vi "Write Log File.vi"(6 "time":dbl format="%.3fs", 7 "error? (F)":bool, 8 "error in (no error)":errorcluster, 9 "line text":string, 10 "line tag":string, 11 "file refnum in":refnum<file>) -> (0 "error out":errorcluster, 3 "file refnum out":refnum<file>)   [LabVIEW 2017, in "DSF Core.lvlib" / "Logging Thread.lvclass"]
uses:
  Logging Thread.lvclass
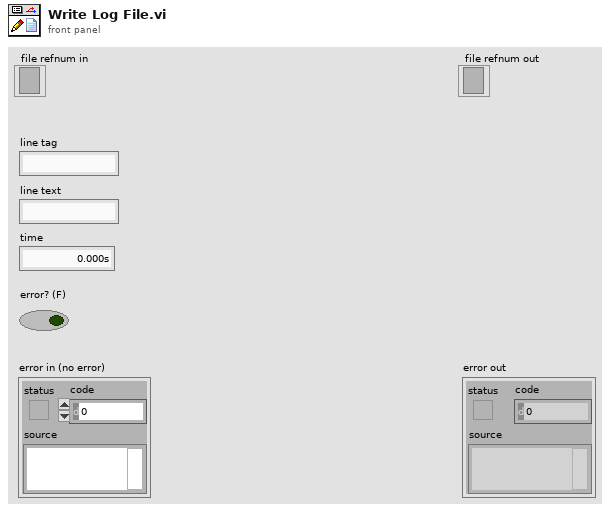
[diagram p1: front panel]
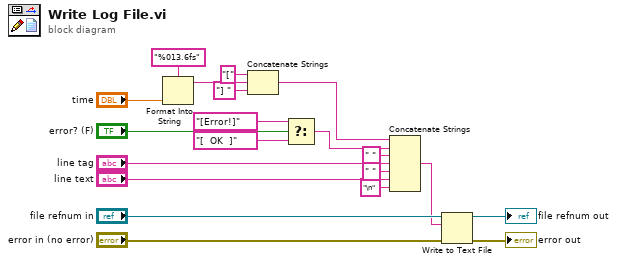
[diagram p0: block diagram]
diagram:
  n1 = Format Into String(format string="%013.6fs", "time") -> (resulting string=w7:string)  [unwired: 2 in, 1 out]
  n2 = Concatenate Strings("[" ("string"), w7, "] " ("string")) -> (w3:string)
  n3 = Select(t="[Error!]", s="error? (F)", f="[  OK  ]") -> (s? t:f=w2:string)
  n4 = Concatenate Strings(w3, w2, " " ("string"), "line tag", " " ("string"), "line text", "\n" ("string")) -> (w16:string)
  n5 = Write to Text File(file (use dialog)="file refnum in", text=w16, error in="error in (no error)") -> (refnum out=→"file refnum out":refnum<file>, error out=→"error out":errorcluster)  [unwired: 1 in, 1 out]
